vi "Circus Config Param.vi"(8 "error in (no error)":errorcluster, 11 "Parameter Name":string) -> (0 "error out":errorcluster, 3 "Value":string)   [LabVIEW 2026, in "TALOS.lvlib"]
doc: "Use this VI to access the values of the parameters of the AEgIS_Param.ini."
uses:
  TALOS.lvlib
  Ancestor/Ancestor/Ancestor.lvclass/Ancestor.ctl
  Generate Error.vi
  Circus Root Path.vi
  TALOS Config Param.vi
  FGV/Error Memory/Get Error Description.vi
  Get PC name.vi
  Ancestor/Ancestor/Read ID.vi
  Get Class Name.vi
  <vilib>/Utility/error.llb/Clear Errors.vi
  FGV/Error Memory/Error Memory Core.vi
  <vilib>/AdvancedString/Delimited String to 1D String Array.vi
  <vilib>/AdvancedString/Delimited String to 1D String Array (string).vi
  FGV/Error Memory/Error Crt Lvl checker.vi
  FGV/Error Memory/Error Memory Core.vi/40c8088d-b597-4017-91af-faa98e00292e.vi
  FGV/Error Memory/Error Memory Core.vi/d4a3ab98-063c-4e44-b43d-fbdcfe6c2be2.vi
  Global Memory.vi
  <vilib>/Utility/LVClass/Get LV Class Name.vi
  Is in Packed Library.vi
  TALOS Root path.vi
  Read CSV worksheet.vi
  Global Constants.vi
  <vilib>/Utility/error.llb/General Error Handler.vi
  <vilib>/Utility/config.llb/Open Config Data.vi
  <vilib>/Utility/config.llb/Get Section Names.vi
  <vilib>/Utility/config.llb/Get Key Names.vi
  <vilib>/Utility/config.llb/Read Key.vi
  <vilib>/Utility/config.llb/Read Key (String).vi
  <vilib>/Utility/config.llb/Close Config Data.vi
  Ancestor/Ancestor/Ancestor.lvclass
  <vilib>/Comparison/Equal/Equal Functor/Equal Functor.lvclass
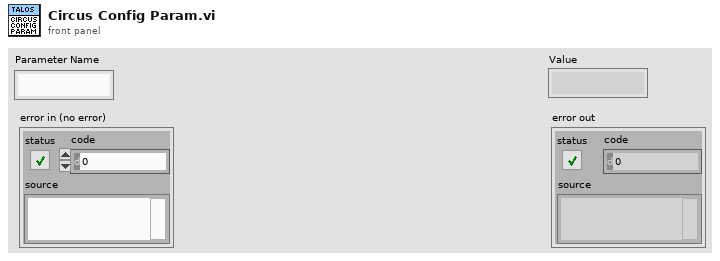
[diagram p1: front panel]
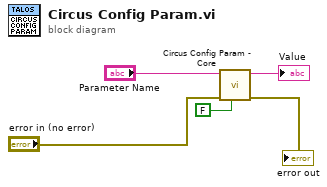
[diagram p0: block diagram]
diagram:
  n1 = call "Circus Config Param - Core.vi"("Load"=FALSE, "error in (no error)"="error in (no error)", "Parameter Name"="Parameter Name") -> ("error out"=→"error out":errorcluster, "Output"=→"Value":string)  [unwired: 7 in]
